vi "ME_acquire_8.vi"() -> ()   [LabVIEW 2015]
doc: "Use this template to build a producer/consumer design pattern. Use this template when you need to execute a process, such as data analysis, when a data source, such as a triggered acquisition, produces data at an uneven rate and you need to execute the process when the data becomes available."
uses:
  Mode.ctl
  oxford_driver/Oxford Drivers/BUSGEN.LLB/OxfordAddress.ctl
  <vilib>/Analysis/baseanly.llb/Mean (DBL).vi
  <vilib>/Utility/file.llb/Write Delimited Spreadsheet (DBL).vi
  <vilib>/express/express arith-compare/Formula/XNode/ExpressFormulaBlockNode.xnode
  <vilib>/Analysis/NI_AALBase.lvlib
panel:
  in  "Target Cnt":i8
  in  "Stop":bool
  out "SaveSweep":bool=TRUE
  out "Measurement File_dn":path
  out "Measurement File_up":path
  out "Measurement File_average":path
  out "Actual Polarization":dbl
  in  "Reset IB?":bool
  in  "First?":bool
  in  "Save Period":dbl=1.0
  out "Averaged I(B)":dbl[][](array[numeric])
  out "P(uC/mm^2)":dbl[](array[numeric])
  in  "Sweep Field":bool
  out "P(B)":cluster{"yi":dbl[], dbl[]}(graph)
  out "Offset array":dbl[](array[numeric])
  in  "stop 2":bool
  in  "dB":dbl=0.005
  in  "Dwell Time (ms)":u32=1
  out "appended array":dbl[][](array[numeric])
  in  "Magnet ON?":bool
  out "Actual B Field (T)":dbl
  out "Actual Temperature (K)":dbl
  out "Actual Current (pA)":dbl
  in  "Tab Control":T1(tab)
  out "P(T)":cluster{"yi":dbl[], dbl[]}(graph)
  out "I(T)":cluster{dbl[], dbl[]}(graph)
  in  "Set temperature (K)":dbl=4.5
  in  "Temp Ramping Rate (K/min)":dbl=10.0
  in  "Heater Range":enum16{"Off", "Low", "Medium", "High"}(ring)
  in  "Heater On/Off":bool
  in  "Sweep Rate Array":dbl[](array[numeric])=[2.0, 1.0, 0.5, 0.1, 0.05, 9.0, 10.0, 11.0, 12.0]
  out "I(B) 3":cluster{dbl[], dbl[]}[](graph)
  in  "Go to Set":bool
  in  "Set Field (T)":dbl=0.3
  in  "Field To Zero":bool
  in  "Sweep Rate (T/min)":dbl=2.0 format="%.6f"
  in  "Min Field (T)":dbl
  in  "Max Field (T)":dbl
  out "Up/Down":bool
  out "I(B) /Averaged/ 2":cluster{"B array":dbl[], dbl[]}[](graph)
  in  "Temperature Array":dbl[](array[numeric])=[4.5, 5.0, 6.0, 7.0, 8.0, 9.0, 10.0, 11.0, 12.0]
  in  "Measure Noise":bool
  in  "Cycles":i32
  in  "maximum value":dbl=10.0 format="%0.2f"
  in  "minimum value":dbl=-10.0 format="%0.2f"
  in  "physical channels":tag="Dev1/ai1"
  out "PSD (pA/Hz^1/2) Peaks Removed":cluster{"f0":dbl, "df":dbl, "magnitude":dbl[]}(graph)
  out "PSD (pA/Hz^1/2)":cluster{"f0":dbl, "df":dbl, "magnitude":dbl[]}(graph)
  out "Current (pA) Filtered":waveform(dbl)(graph)
  out "Current (pA)":dbl[](graph)
  in  "Samples per channel":i32=1000
  in  "Rate":dbl=1000.0 format="%0.2f"
  in  "Cut-Off Frequency":dbl=100.0 caption="Lower Cut-Off"
  in  "Filter On":bool
  out "Dc offset":dbl
  in  "Calibrate":bool
  in  "IV converter":refnum<visa-resource-name>="GPIB0::20::INSTR"
  in  "Magnetic Field":refnum<visa-resource-name>="GPIB0::21::INSTR"
  out "Time Lag":dbl=0.0500025749206543
  in  "Lake Shore":refnum<visa-resource-name>="GPIB0::11::INSTR"
  in  "Temp Refresh (s)":dbl=1.0
  in  "Sampling rate (Hz)":dbl=10.0
  in  "Gain (V/A)":dbl=1000000000.0
  in  "Sample area (mm^2)":dbl=3.9
  out "B_V":cluster{dbl[], "Best Linear Fit":dbl[]}[](graph)=[{[-0.00854253601, 0.00626134724, 0.0219834428, 0.0379117736, 0.0535871506, 0.0694316728, 0.0851615152, 0.100816481, 0.116478038, 0.132148461, 0.147876163, 0.16341701, 0.178976744, 0.194563632, 0.210251739, 0.225738944, 0.241298253, 0.256806034, 0.272344374, 0.287933477, 0.303494709, 0.318997125, 0.334591297, 0.350146681, 0.365618053, 0.380940961, 0.39666457, 0.412213675, 0.427724671, 0.443221444, 0.458760641, 0.474360042, 0.489915118, 0.505330598, 0.520967119, 0.536347531, 0.551813711, 0.567441155, 0.582995861, 0.598507522, 0.614041988, 0.629563151, 0.645106262, 0.660611914, 0.676136149, 0.691553948, 0.7071244, 0.72262999, 0.738171137, 0.753700392, 0.76919513, 0.784778028, 0.800215944, 0.8156961, 0.831325434, 0.846852183, 0.862326812, 0.877819169, 0.893312568, 0.90888536, 0.924354789], "Best Linear Fit"=[0.0, 0.005, 0.01, 0.015, 0.02, 0.025, 0.03, 0.035, 0.04, 0.045, 0.05, 0.055, 0.06, 0.065, 0.07, 0.075, 0.08, 0.085, 0.09, 0.095, 0.1, 0.105, 0.11, 0.115, 0.12, 0.125, 0.13, 0.135, 0.14, 0.145, 0.15, 0.155, 0.16, 0.165, 0.17, 0.175, 0.18, 0.185, 0.19, 0.195, 0.2, 0.205, 0.21, 0.215, 0.22, 0.225, 0.23, 0.235, 0.24, 0.245, 0.25, 0.255, 0.26, 0.265, 0.27, 0.275, 0.28, 0.285, 0.29, 0.295, 0.3]}, {[-0.00854253601, 0.00626134724, 0.0219834428, 0.0379117736, 0.0535871506, 0.0694316728, 0.0851615152, 0.100816481, 0.116478038, 0.132148461, 0.147876163, 0.16341701, 0.178976744, 0.194563632, 0.210251739, 0.225738944, 0.241298253, 0.256806034, 0.272344374, 0.287933477, 0.303494709, 0.318997125, 0.334591297, 0.350146681, 0.365618053, 0.380940961, 0.39666457, 0.412213675, 0.427724671, 0.443221444, 0.458760641, 0.474360042, 0.489915118, 0.505330598, 0.520967119, 0.536347531, 0.551813711, 0.567441155, 0.582995861, 0.598507522, 0.614041988, 0.629563151, 0.645106262, 0.660611914, 0.676136149, 0.691553948, 0.7071244, 0.72262999, 0.738171137, 0.753700392, 0.76919513, 0.784778028, 0.800215944, 0.8156961, 0.831325434, 0.846852183, 0.862326812, 0.877819169, 0.893312568, 0.90888536, 0.924354789], "Best Linear Fit"=[-0.00022554388023060128, 0.004536267537808887, 0.009593430775915074, 0.014716931562355689, 0.01975906732634002, 0.024855610270593523, 0.029915265354287977, 0.03495083565949541, 0.03998852608757118, 0.045029068349812316, 0.05008803495326229, 0.055086897848955874, 0.060091835929837946, 0.06510550835596321, 0.07015173884687344, 0.07513334727738563, 0.08013814865293042, 0.08512637555172443, 0.0901244320467579, 0.09513881694893507, 0.10014423687592358, 0.10513073807087174, 0.11014675346564809, 0.1151502923271957, 0.12012680792099008, 0.1250555686413888, 0.1301132186920259, 0.13511473785283767, 0.14010399888730068, 0.14508868495702945, 0.1500870171143548, 0.15510471446726903, 0.16010815425765457, 0.16506669165212906, 0.17009632901003072, 0.1750435864450521, 0.18001843198211442, 0.1850451496356715, 0.19004847041199868, 0.1950379453501071, 0.20003475573578386, 0.20502728708357412, 0.21002687821664084, 0.21501442030211, 0.220007939788244, 0.2249672231113706, 0.22997560874002893, 0.23496313088260184, 0.23996209027618054, 0.24495722449359253, 0.24994125598600042, 0.2549536449902534, 0.25991939913989753, 0.2648987401917687, 0.26992606578200207, 0.2749203939204135, 0.2798979571595809, 0.2848812227804405, 0.2898648235706211, 0.2948739618827834, 0.2998498524919418]}]
  out "V_I":cluster{dbl[], "Best Linear Fit":dbl[]}[](graph)=[{[0.0, 0.035, 0.069, 0.104, 0.138, 0.173, 0.208, 0.242, 0.277, 0.311, 0.346, 0.38, 0.415, 0.45, 0.484, 0.519, 0.553, 0.588, 0.623, 0.657, 0.692, 0.726, 0.761, 0.796, 0.83, 0.865, 0.899, 0.934, 0.969, 1.003, 1.038, 1.072, 1.107, 1.141, 1.176, 1.211, 1.245, 1.28, 1.314, 1.349, 1.384, 1.418, 1.453, 1.487, 1.522, 1.557, 1.591, 1.626, 1.66, 1.695, 1.73, 1.764, 1.799, 1.833, 1.868, 1.902, 1.937, 1.972, 2.006, 2.041, 2.075], "Best Linear Fit"=[-0.00854253601, 0.00626134724, 0.0219834428, 0.0379117736, 0.0535871506, 0.0694316728, 0.0851615152, 0.100816481, 0.116478038, 0.132148461, 0.147876163, 0.16341701, 0.178976744, 0.194563632, 0.210251739, 0.225738944, 0.241298253, 0.256806034, 0.272344374, 0.287933477, 0.303494709, 0.318997125, 0.334591297, 0.350146681, 0.365618053, 0.380940961, 0.39666457, 0.412213675, 0.427724671, 0.443221444, 0.458760641, 0.474360042, 0.489915118, 0.505330598, 0.520967119, 0.536347531, 0.551813711, 0.567441155, 0.582995861, 0.598507522, 0.614041988, 0.629563151, 0.645106262, 0.660611914, 0.676136149, 0.691553948, 0.7071244, 0.72262999, 0.738171137, 0.753700392, 0.76919513, 0.784778028, 0.800215944, 0.8156961, 0.831325434, 0.846852183, 0.862326812, 0.877819169, 0.893312568, 0.90888536, 0.924354789]}, {[0.0, 0.035, 0.069, 0.104, 0.138, 0.173, 0.208, 0.242, 0.277, 0.311, 0.346, 0.38, 0.415, 0.45, 0.484, 0.519, 0.553, 0.588, 0.623, 0.657, 0.692, 0.726, 0.761, 0.796, 0.83, 0.865, 0.899, 0.934, 0.969, 1.003, 1.038, 1.072, 1.107, 1.141, 1.176, 1.211, 1.245, 1.28, 1.314, 1.349, 1.384, 1.418, 1.453, 1.487, 1.522, 1.557, 1.591, 1.626, 1.66, 1.695, 1.73, 1.764, 1.799, 1.833, 1.868, 1.902, 1.937, 1.972, 2.006, 2.041, 2.075], "Best Linear Fit"=[-0.007846580254753975, 0.007882153481927697, 0.02316149482613275, 0.03889022856281441, 0.054169569907019474, 0.06989830364370113, 0.08562703738038281, 0.10090637872458785, 0.11663511246126955, 0.1319144538054746, 0.14764318754215625, 0.1629225288863613, 0.17865126262304296, 0.19437999635972467, 0.2096593377039297, 0.22538807144061138, 0.24066741278481643, 0.25639614652149806, 0.27212488025817977, 0.2874042216023848, 0.3031329553390665, 0.31841229668327153, 0.3341410304199532, 0.3498697641566349, 0.3651491055008399, 0.3808778392375216, 0.39615718058172666, 0.4118859143184083, 0.42761464805509, 0.442893989399295, 0.45862272313597674, 0.4739020644801818, 0.48963079821686345, 0.5049101395610684, 0.5206388732977502, 0.5363676070344319, 0.5516469483786369, 0.5673756821153185, 0.5826550234595236, 0.5983837571962053, 0.6141124909328869, 0.629391832277092, 0.6451205660137737, 0.6603999073579787, 0.6761286410946604, 0.691857374831342, 0.7071367161755471, 0.7228654499122288, 0.7381447912564338, 0.7538735249931156, 0.7696022587297972, 0.7848816000740022, 0.8006103338106839, 0.815889675154889, 0.8316184088915707, 0.8468977502357756, 0.8626264839724573, 0.878355217709139, 0.893634559053344, 0.9093632927900257, 0.9246426341342309]}]
  out "B0 (T)":dbl=0.0025222449819540214
  out "B/V (T/V)":dbl=0.321659617116981
  out "I0 (A)":dbl=-0.007846580254753975
  out "V/I (Ohm)":dbl=0.44939239247661916
  in  "Offset?":bool
  in  "Temp/Magnetic Field":bool
  out "index":i8
  out "Read?":bool
  out "Magnetic Field (T)":dbl[](array[numeric])
  out "Reset":bool
  out "Measured Current (pA)":dbl[](array[numeric])
  out "Elapsed Time (s)":dbl[](array[numeric])
  out "Start time":timestamp
  in  "Enum":T2=enum."Process"
  out "B array":dbl[](array[numeric])
  in  "dB (T)":dbl=0.005
  in  "Counter":i8
  out "L magnet (H)":dbl
  out "R magnet (mOhm)":dbl
  out "Actual Current (R0)":dbl
  out "Actual Field (T)":dbl
  out "Temperature array":dbl[](array[numeric])
  in  "New Measurement File":bool
  out "Measurement File":path
  out "refnum out":refnum<file>
  in  "Measuring":bool
  in  "Measure /Pause":bool
  in  "stop":bool
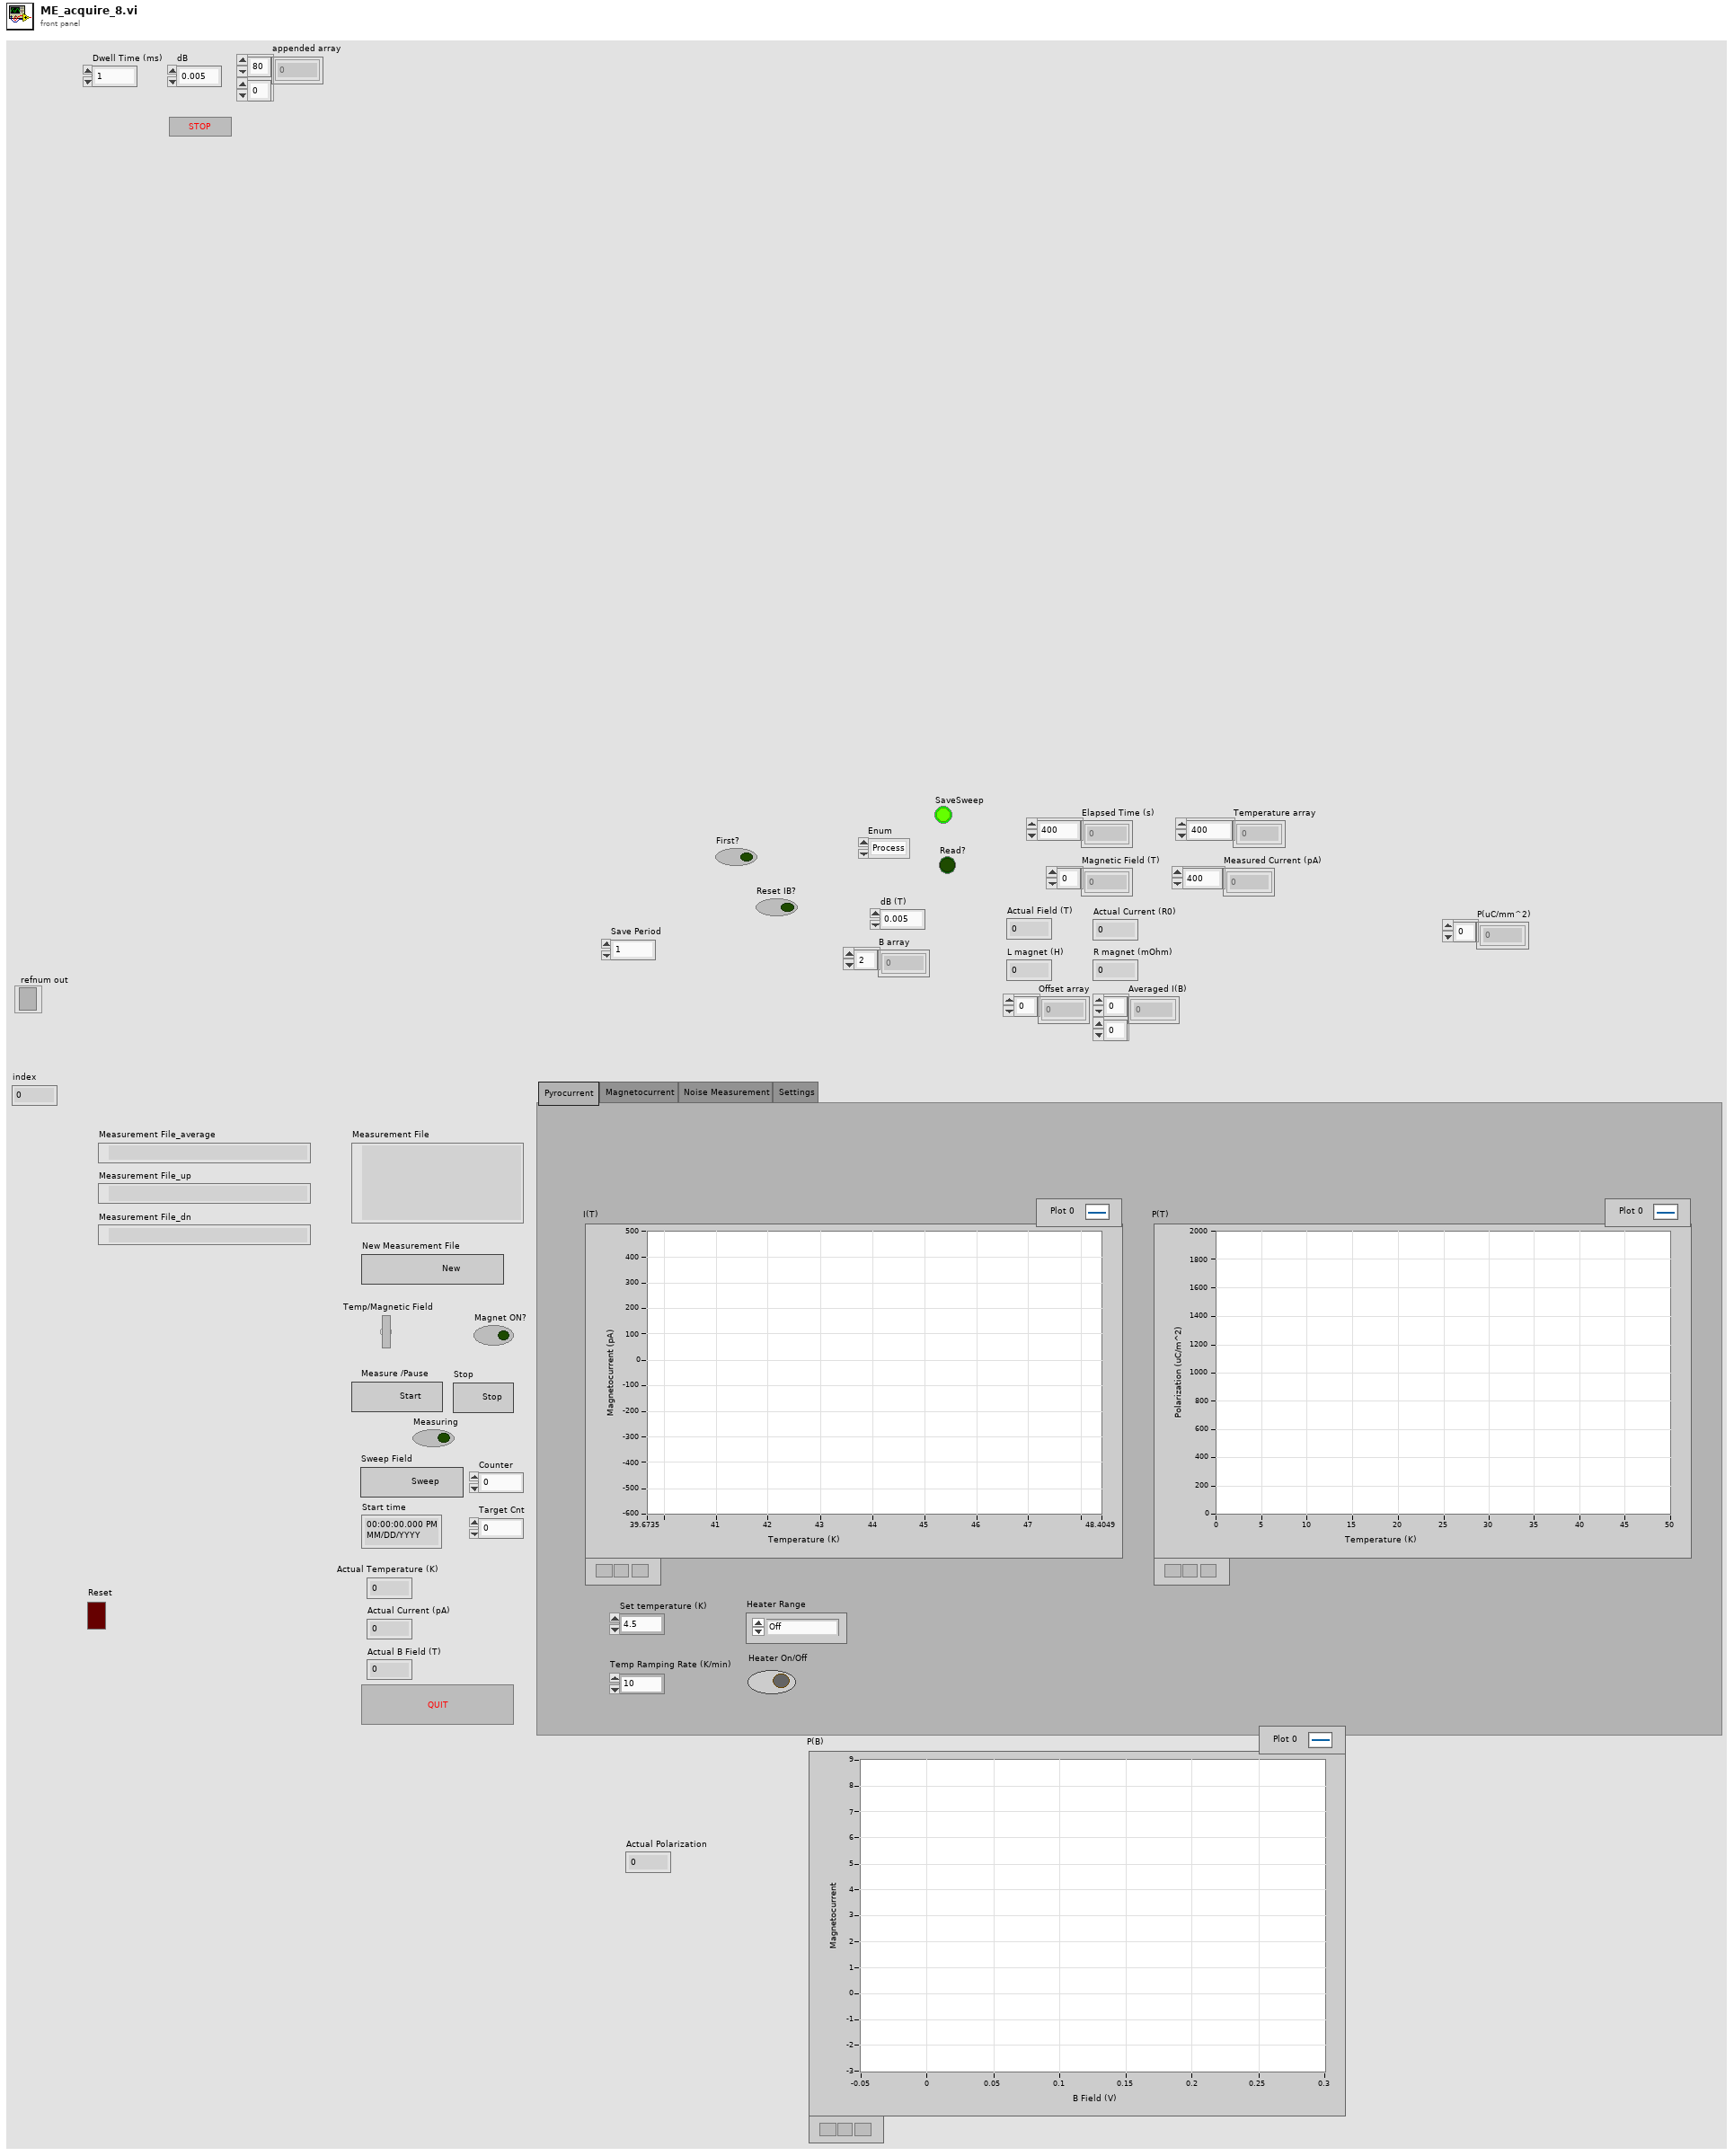
[diagram p1: front panel]
types:
  T1 = enum32{"Pyrocurrent", "Magnetocurrent", "Noise Measurement", "Settings"}
  T2 = typedef "Mode.ctl" = enum16{"Offset", "Process", "Sweep", "Plot", "Save", "New"}
  T3 = enum16{"open", "replace", "create", "open or create", "replace or create", "replace or create with confirmation"}
  T4 = typedef "OxfordAddress.ctl" = cluster{"Com Port":i32, "ISOBUS Address":i32, "GPIB Address":i16, "Communication":enum16{"RS232", "ISOBUS", "GPIB", "Gateway"}}
  T5 = cluster{"seconds since 1Jan1904":timestamp, "read buffer":string, "read buffer":string}
  T6 = cluster{"B array":dbl[], "Averaged I(B) out":dbl[]}
  T7 = cluster{"B array":dbl[], "Averaged I(B) out":dbl[]}[]
  T8 = cluster{"I array out (A)":dbl[], "V array out (V)":dbl[]}
  T9 = cluster{"I array out (A)":dbl[], "Best Linear Fit":dbl[]}
  T10 = cluster{"V array out (V)":dbl[], "B array Out":dbl[]}
  T11 = cluster{"V array out (V)":dbl[], "Best Linear Fit 2":dbl[]}
  T12 = cluster{"I array out (A)":dbl[], "Best Linear Fit":dbl[]}[]
  T13 = cluster{"V array out (V)":dbl[], "Best Linear Fit 2":dbl[]}[]
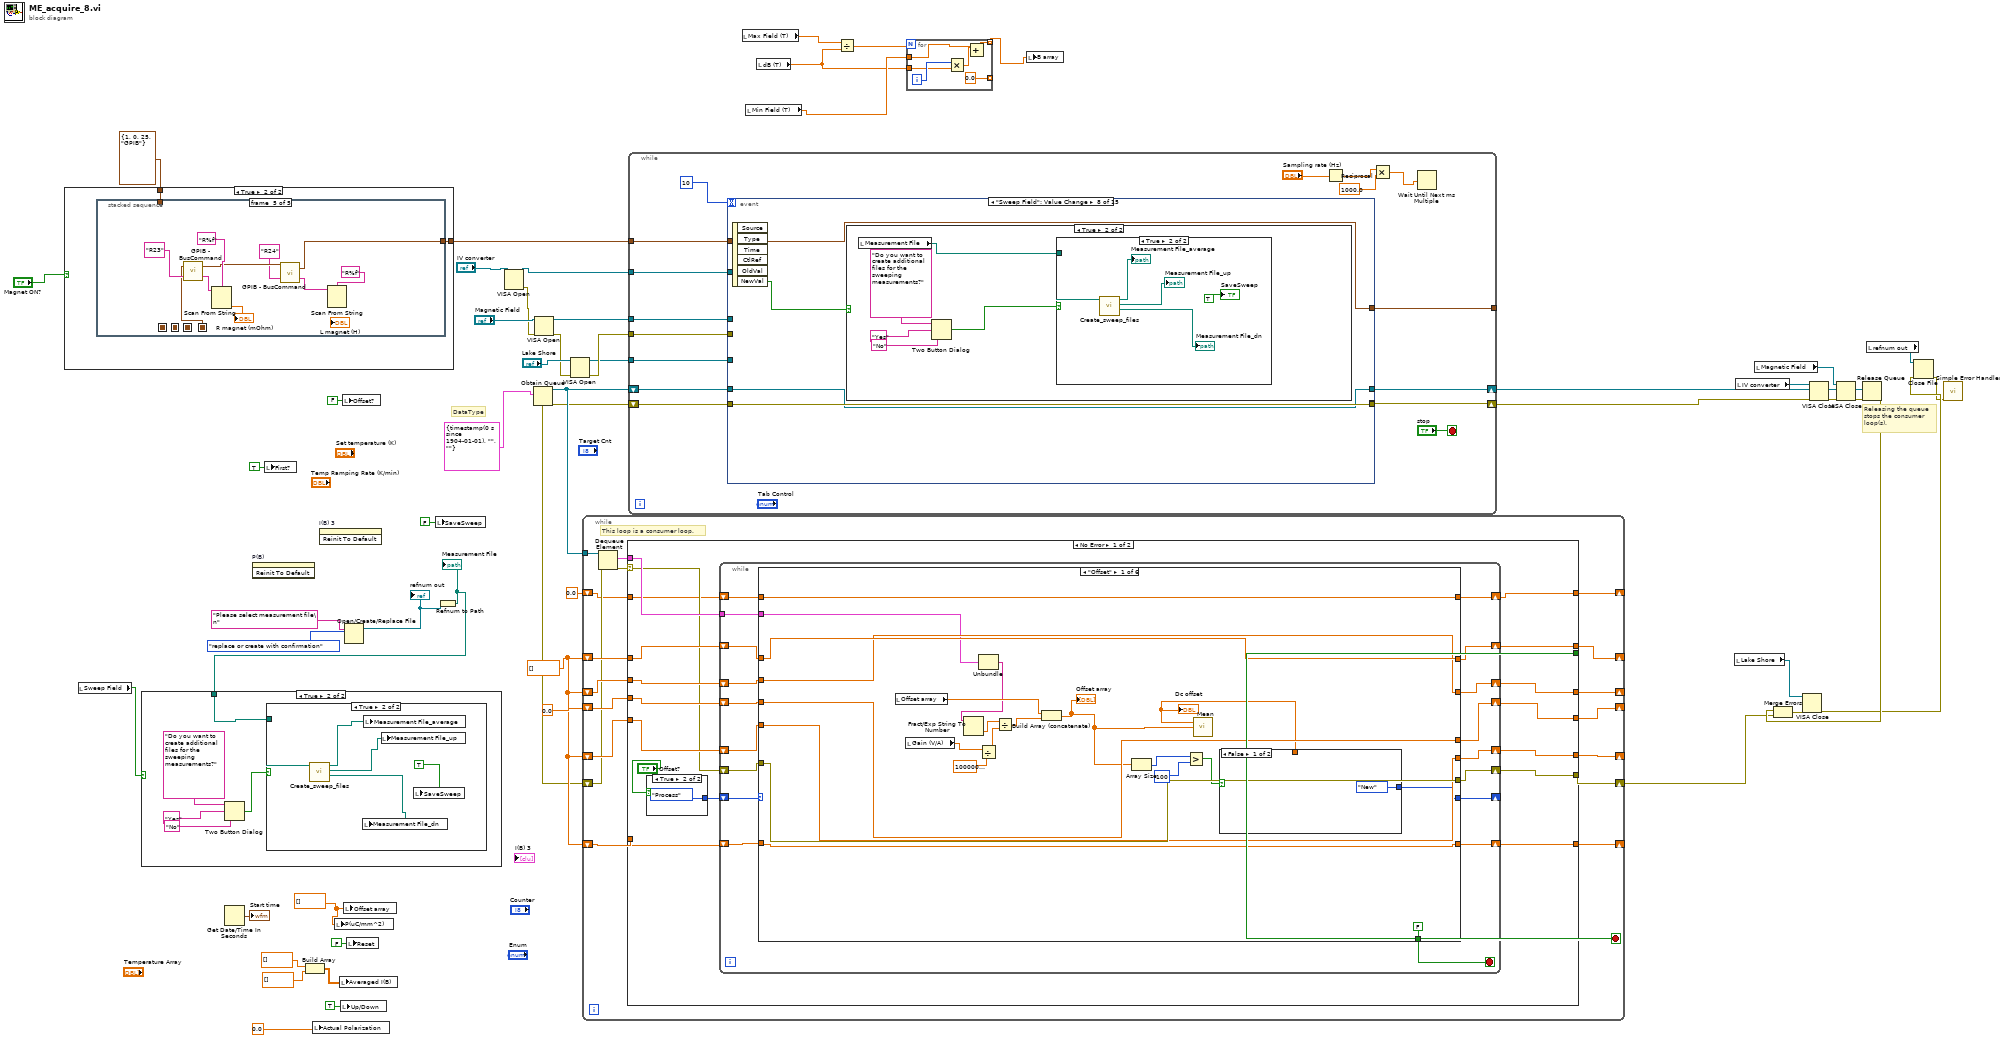
[diagram p0: block diagram]
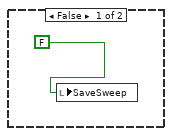
[diagram p3: hidden frame]
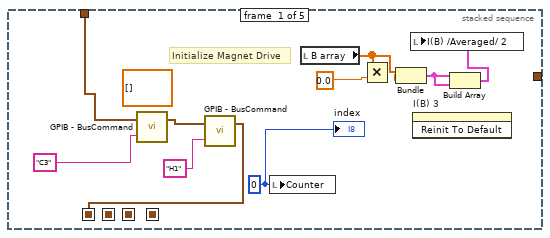
[diagram p5: hidden frame]
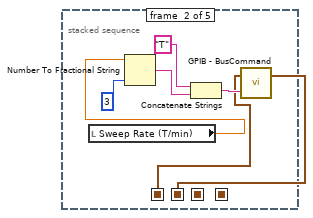
[diagram p6: hidden frame]
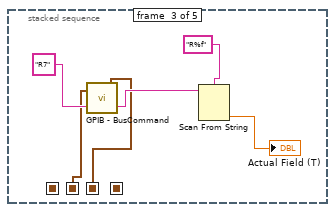
[diagram p7: hidden frame]
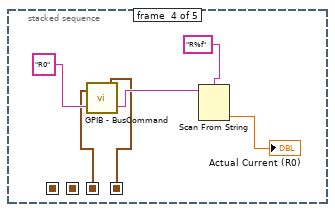
[diagram p8: hidden frame]
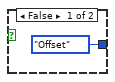
[diagram p9: hidden frame]
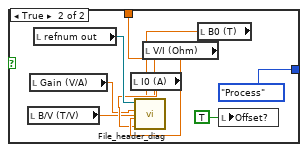
[diagram p10: hidden frame]
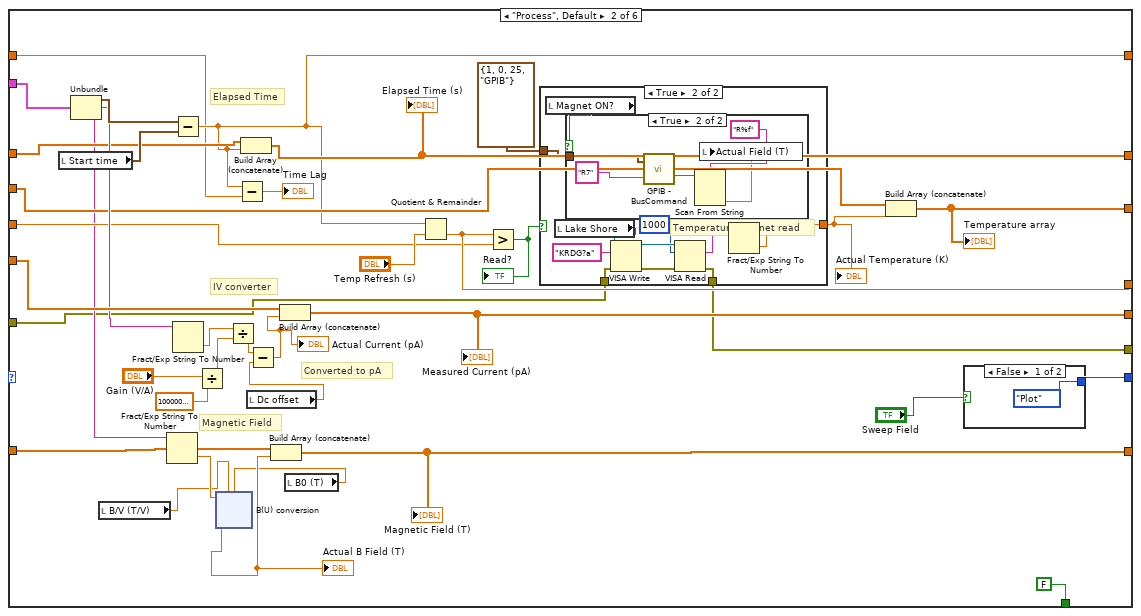
[diagram p11: hidden frame]
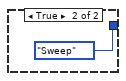
[diagram p12: hidden frame]
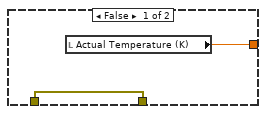
[diagram p13: hidden frame]
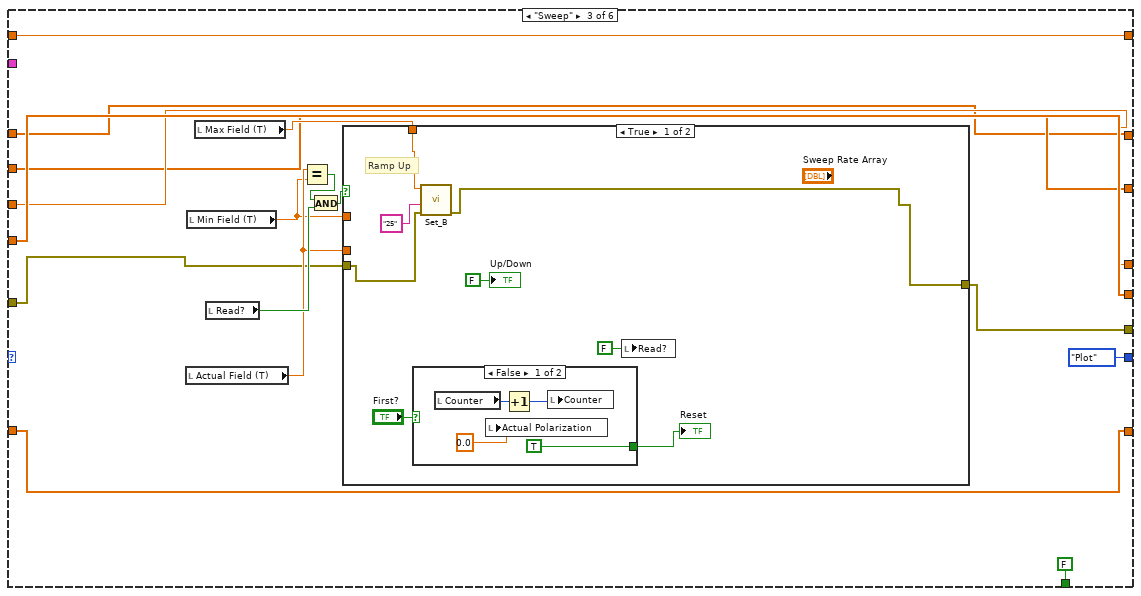
[diagram p15: hidden frame]
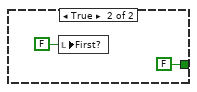
[diagram p16: hidden frame]
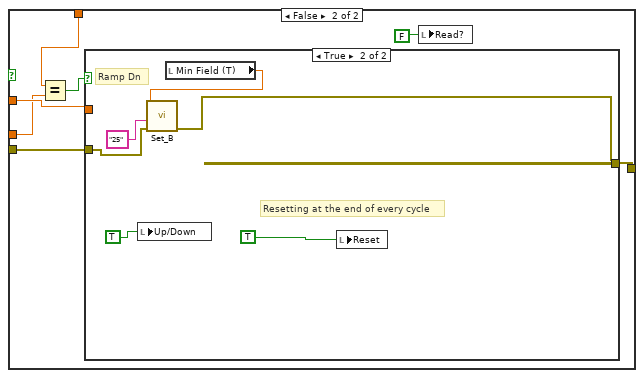
[diagram p17: hidden frame]
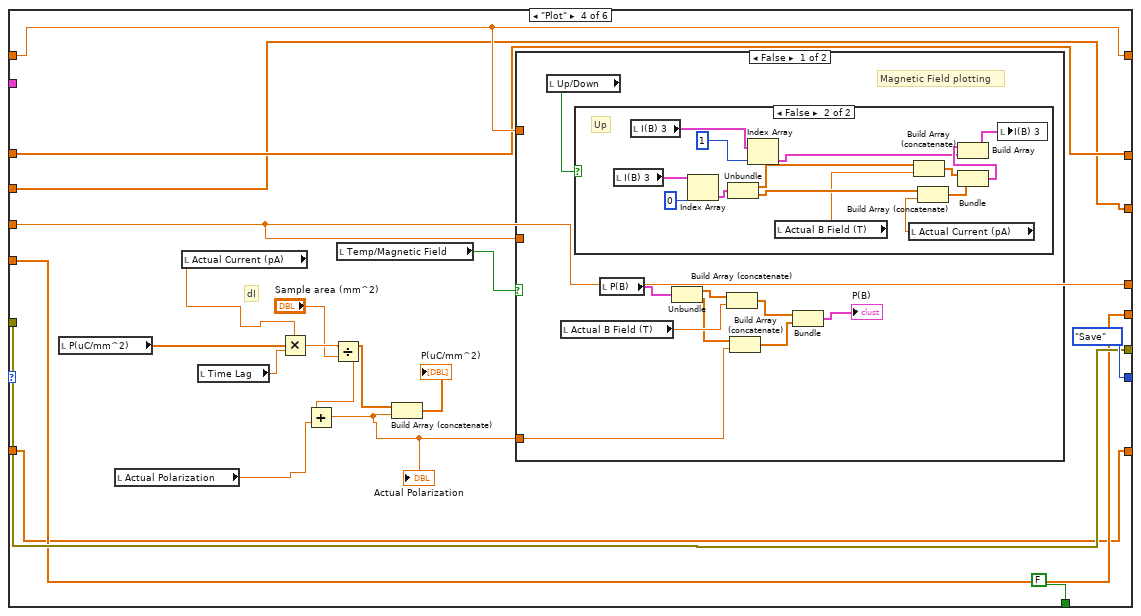
[diagram p19: hidden frame]
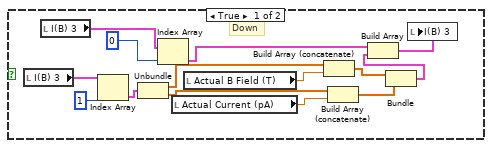
[diagram p20: hidden frame]
diagram:
  w16 = dbl[] []
  w23 = dbl[] []
  # "DataType"
  # "Releasing the queue stops the consumer loop(s)."
  n1 = case shown="True" "Magnet ON?" {
    tunnel: T4 {"Com Port"=1, "ISOBUS Address"=0, "GPIB Address"=25, "Communication"=enum."GPIB"} ("Address") -> [w53 w55]
    tunnel: [w53 w54] -> w31
    frame False {
    }
    frame True {
      n2 = stacked-sequence {
        seq-local: [w63 _ _ _ _] -> [_ w68 _ _ _]
        seq-local: [_ w67 _ _ _] -> [_ _ w75 _ _]
        seq-local: [_ _ w74 _ _] -> [_ _ _ w81 _]
        seq-local: [_ _ _ w80 _] -> [_ _ _ _ w91]
        tunnel: w55 -> [w65 _ _ _ _]
        tunnel: [_ _ _ _ w89] -> w54
        frame #0 {
          (unwired) dbl[][] []
          w61 = i8 0 ("Counter")
          # "Initialize Magnet Drive"
          n3 = call "GPIB - BusCommand.vi"("Command"="C3", "Address"=w65) -> ("Address(thru)"=w64:T4)  [unwired: 1 out]
          n4 = call "GPIB - BusCommand.vi"("Command"="H1", "Address"=w64) -> ("Address(thru)"=w63:T4)  [unwired: 1 out]
          n5 = local write "Counter"(w61) -> ()
          n6 = local read "B array"() -> (w59:dbl[])
          n7 = Multiply(x=w59, y=0.0) -> (x*y=w58:dbl[])
          n8 = Bundle("B array"=w59, w58) -> (w57:cluster{"B array":dbl[], dbl[]})  [unwired: 1 in]
          n9 = invoke on="I(B) 3" class="XYGraph (strict)" method="Reinit To Default"() -> ()  [unwired: 3 in, 3 out]
          n10 = Build Array(w57, w57) -> (w56:cluster{"B array":dbl[], dbl[]}[])
          n11 = local write "I(B) /Averaged/ 2"(w56) -> ()
          "index" <- w61
        }
        frame #1 {
          n12 = local read "Sweep Rate (T/min)"() -> (w69:dbl)
          n13 = Number To Fractional String(number=w69, precision (6)=i16 3) -> (F-format string=w71:string)  [unwired: 2 in]
          n14 = Concatenate Strings("T" ("format string"), w71) -> (w70:string)
          n15 = call "GPIB - BusCommand.vi"("Command"=w70, "Address"=w68) -> ("Address(thru)"=w67:T4)  [unwired: 1 out]
        }
        frame #2 {
          n16 = call "GPIB - BusCommand.vi"("Command"="R7" ("format string"), "Address"=w75) -> ("Reply"=w79:string, "Address(thru)"=w74:T4)
          n17 = Scan From String(format string="R%f" ("remaining string"), input string=w79) -> (output 1=→"Actual Field (T)":dbl)  [unwired: 3 in, 3 out]
        }
        frame #3 {
          n18 = call "GPIB - BusCommand.vi"("Command"="R0" ("format string"), "Address"=w81) -> ("Reply"=w85:string, "Address(thru)"=w80:T4)
          n19 = Scan From String(format string="R%f" ("remaining string"), input string=w85) -> (output 1=→"Actual Current (R0)":dbl)  [unwired: 3 in, 3 out]
        }
        frame #4 {
          n20 = call "GPIB - BusCommand.vi"("Command"="R23" ("format string"), "Address"=w91) -> ("Reply"=w95:string, "Address(thru)"=w90:T4)
          n21 = Scan From String(format string="R%f" ("remaining string"), input string=w95) -> (output 1=→"R magnet (mOhm)":dbl)  [unwired: 3 in, 3 out]
          n22 = call "GPIB - BusCommand.vi"("Command"="R24" ("format string"), "Address"=w90) -> ("Reply"=w87:string, "Address(thru)"=w89:T4)
          n23 = Scan From String(format string="R%f" ("remaining string"), input string=w87) -> ()  [unwired: 4 in, 3 out]
        }
      }
    }
  }
  n24 = local read "Sweep Field"() -> (w2:bool)
  n25 = Get Date/Time In Seconds() -> (seconds since 1Jan1904=→"Start time":timestamp)
  n26 = invoke on="P(B)" class="XYGraph (strict)" method="Reinit To Default"() -> ()  [unwired: 3 in, 3 out]
  n27 = local write "First?"(TRUE ("First?")) -> ()
  n28 = Build Array(dbl[] [], dbl[] []) -> (w13:dbl[][])
  n29 = local write "Actual Polarization"(0.0 ("Actual Polarization")) -> ()
  n30 = invoke on="I(B) 3" class="XYGraph (strict)" method="Reinit To Default"() -> ()  [unwired: 3 in, 3 out]
  n31 = local write "P(uC/mm^2)"(w16) -> ()
  n32 = local write "Averaged I(B)"(w13) -> ()
  n33 = local write "Up/Down"(TRUE ("Up/Down")) -> ()
  n34 = local write "Offset?"(FALSE ("Offset?")) -> ()
  n35 = local write "Offset array"(w16) -> ()
  n36 = Open/Create/Replace File(prompt="Please select measurement file\n", operation (0:open)=T3."replace or create with confirmation") -> (refnum out=w28:refnum<file>)  [unwired: 4 in, 2 out]
  "refnum out" <- w28
  n37 = local write "Reset"(FALSE ("Reset")) -> ()
  n38 = local write "SaveSweep"(FALSE ("SaveSweep")) -> ()
  n39 = Refnum to Path(1:w28) -> (0:w1:path)
  "Measurement File" <- w1
  n40 = case shown="True" w2 {
    tunnel: w1 -> [_ w96]
    frame False {
    }
    frame True {
      n41 = Two Button Dialog(message="Do you want to create additional files for the sweeping measurements?" ("string"), 1:"No" ("F button name (\"Cancel\")"), 2:"Yes" ("T button name (\"OK\")")) -> (T button?=w98:bool)
      n42 = case shown="True" w98 {
        tunnel: w96 -> [_ w106]
        frame False {
          n43 = local write "SaveSweep"(FALSE ("SaveSweep")) -> ()
        }
        frame True {
          n44 = call "Create_sweep_files.vi"("Measurement File"=w106) -> ("Path 3"=w103:path, "Path 2"=w104:path, "Path"=w105:path)  [unwired: 8 in]
          n45 = local write "Measurement File_dn"(w103) -> ()
          n46 = local write "Measurement File_average"(w105) -> ()
          n47 = local write "Measurement File_up"(w104) -> ()
          n48 = local write "SaveSweep"(TRUE) -> ()
        }
      }
    }
  }
  n49 = VISA Open(VISA resource name="IV converter") -> (VISA resource name=w47:refnum<visa-resource-name>, error out=w49:errorcluster)  [unwired: 4 in]
  n50 = Obtain Queue(element data type=T5 {"seconds since 1Jan1904"=timestamp(0 s since 1904-01-01), "read buffer"="", "read buffer"=""} ("output cluster")) -> (queue out=w52:refnum<queue>, error out=w21:errorcluster)  [unwired: 4 in, 1 out]
  n51 = VISA Open(error in (no error)=w49, VISA resource name="Magnetic Field") -> (VISA resource name=w46:refnum<visa-resource-name>, error out=w25:errorcluster)  [unwired: 3 in]
  n52 = VISA Open(error in (no error)=w25, VISA resource name="Lake Shore") -> (VISA resource name=w19:refnum<visa-resource-name>, error out=w24:errorcluster)  [unwired: 3 in]
  n53 = while {
    tunnel: w52 -> [w124]
    shift-right: [w119] -> _
    shift-left: w23 -> [w118]
    shift-right: [w117] -> _
    shift-left: w23 -> [w116]
    shift-right: [w115] -> _
    shift-left: w23 -> [w114]
    shift-right: [w113] -> _
    shift-left: 0.0 -> [w112]
    shift-right: [w111] -> _
    shift-left: w23 -> [w110]
    shift-right: [w120] -> w36
    shift-left: w21 -> [w109]
    shift-right: [w108] -> _
    shift-left: 0.0 -> [w107]
    stop <- w121 stop-if-true
    # "This loop is a consumer loop."
    n54 = Dequeue Element(queue=w124, error in (no error)=w109) -> (element=w122:T5, error out=w123:errorcluster)  [unwired: 1 in, 2 out]
    n55 = case shown="No Error" w123 {
      selector: w123 -> [w129 w462]
      tunnel: w122 -> [w140 _]
      tunnel: [_ TRUE] -> w121
      tunnel: [w128 w462] -> w120
      tunnel: [w139 w461] -> w119
      tunnel: w118 -> [w138 w461]
      tunnel: [w137 w458] -> w117
      tunnel: w116 -> [w136 w458]
      tunnel: [w135 w457] -> w115
      tunnel: w114 -> [w134 w457]
      tunnel: [w133 w459] -> w113
      tunnel: w112 -> [w132 w459]
      tunnel: [w131 w460] -> w111
      tunnel: w110 -> [w130 w460]
      tunnel: [w127 w456] -> w108
      tunnel: w107 -> [w126 w456]
      frame No Error {
        n56 = case shown="True" "Offset?" {
          tunnel: [Mode."Offset" ("Enum") Mode."Process" ("Enum")] -> w141
          frame False {
          }
          frame True {
          }
        }
        n57 = while {
          shift-right: [w149] -> _
          shift-left: w141 -> [w161]
          tunnel: w140 -> [w160]
          shift-right: [w159] -> w139
          shift-left: w138 -> [w158]
          shift-right: [w151] -> w131
          shift-left: w130 -> [w150]
          shift-right: [w153] -> w133
          shift-left: w132 -> [w152]
          shift-right: [w157] -> w137
          shift-left: w136 -> [w156]
          shift-right: [w147] -> w128
          shift-left: w129 -> [w148]
          shift-right: [w155] -> w135
          shift-left: w134 -> [w154]
          shift-right: [w145] -> w127
          shift-left: w126 -> [w144]
          stop <- w146 stop-if-true
          n58 = case shown="\"Offset\"" w161 {
            tunnel: w160 -> [w176 w229 _ _ _ _]
            tunnel: [w183 w226 w266 w319 w392 w454] -> w159
            tunnel: w158 -> [w183 w217 w266 w319 w388 w454]
            tunnel: [w177 w225 w269 w321 w394 w451] -> w157
            tunnel: w156 -> [w177 w224 w269 w321 w389 w451]
            tunnel: [w179 w221 w271 w316 w395 w448] -> w155
            tunnel: w154 -> [w179 w220 w271 w316 w390 w448]
            tunnel: [w181 w216 w268 w317 w398 w452] -> w153
            tunnel: w152 -> [w181 w215 w268 w317 w398 w452]
            tunnel: [w182 w212 w267 w318 w393 w453] -> w151
            tunnel: w150 -> [w182 w213 w267 w318 w391 w453]
            tunnel: [w165 w210 Mode."Plot" ("Enum") Mode."Save" ("Enum") Mode."New" ("Enum") Mode."Process" ("Enum")] -> w149
            tunnel: w148 -> [w180 w208 w273 w324 w397 w450]
            tunnel: [w180 w207 w272 w324 w397 w450] -> w147
            tunnel: [FALSE FALSE FALSE FALSE FALSE TRUE] -> w146
            tunnel: [w164 w204 w265 w320 w396 w447] -> w145
            tunnel: w144 -> [w164 w203 w265 w320 w396 w447]
            frame "Offset" {
              n59 = local read "Offset array"() -> (w170:dbl[])
              n60 = local read "Gain (V/A)"() -> (w174:dbl)
              n61 = Unbundle(w176) -> ("read buffer"=w163:string)  [unwired: 2 out]
              n62 = Fract/Exp String To Number(string=w163) -> (number=w175:dbl)  [unwired: 3 in, 1 out]
              n63 = Divide(x=w174, y=1000000000000.0) -> (x/y=w172:dbl)
              n64 = Divide(x=w175, y=w172) -> (x/y=w171:dbl)
              n65 = Build Array (concatenate)(w170, w171) -> (w166:dbl[])
              "Offset array" <- w166
              n66 = Array Size(array=w166) -> (size(s)=w169:i32)
              n67 = Greater?(x=w169, y=100) -> (0:w167:bool)
              n68 = call-poly <vilib>:"Mean.vi"("X"=w166) -> ("mean"=w162:dbl)  [unwired: 1 out]
              "Dc offset" <- w162
              n69 = case shown="False" w167 {
                tunnel: [Mode."New" ("Enum") Mode."Process" ("Enum")] -> w165
                tunnel: w162 -> [_ w185]
                frame False {
                }
                frame True {
                  n70 = local read "B/V (T/V)"() -> (w186:dbl)
                  n71 = local read "Gain (V/A)"() -> (w187:dbl)
                  n72 = local read "refnum out"() -> (w191:refnum<file>)
                  n73 = local read "I0 (A)"() -> (w189:dbl)
                  n74 = local read "V/I (Ohm)"() -> (w190:dbl)
                  n75 = local read "B0 (T)"() -> (w188:dbl)
                  n76 = call "File_header_diag.vi"("OFFSET"=w185, "B0"=w188, "B/V"=w186, "I0"=w189, "V/I"=w190, "Gain"=w187, "Byte Stream File in"=w191) -> ()  [unwired: 5 in]
                  n77 = local write "Offset?"(TRUE ("Offset?")) -> ()
                }
              }
            }
            frame "Process", Default {
              # "Converted to pA"
              # "Magnetic Field"
              # "IV converter"
              # "Elapsed Time"
              n78 = local read "Start time"() -> (w227:timestamp)
              n79 = Unbundle(w229) -> ("seconds since 1Jan1904"=w228:timestamp, "read buffer"=w222:string, "read buffer"=w209:string)
              n80 = local read "B/V (T/V)"() -> (w199:dbl)
              n81 = Fract/Exp String To Number(string=w209) -> (number=w219:dbl)  [unwired: 3 in, 1 out]
              n82 = Subtract(x=w228, y=w227) -> (x-y=w204:dbl)
              n83 = Fract/Exp String To Number(string=w222) -> (number=w223:dbl)  [unwired: 3 in, 1 out]
              n84 = Divide(x="Gain (V/A)", y=1000000000000.0) -> (x/y=w202:dbl)
              n85 = Divide(x=w223, y=w202) -> (x/y=w197:dbl)
              n86 = Subtract(x=w204, y=w203) -> (x-y=→"Time Lag":dbl)
              n87 = Build Array (concatenate)(w217, w204) -> (w226:dbl[])
              "Elapsed Time (s)" <- w226
              n88 = local read "Dc offset"() -> (w195:dbl)
              n89 = Subtract(x=w197, y=w195) -> (x-y=w196:dbl)
              "Actual Current (pA)" <- w196
              n90 = Build Array (concatenate)(w224, w196) -> (w225:dbl[])
              "Measured Current (pA)" <- w225
              n91 = local read "B0 (T)"() -> (w198:dbl)
              n92 = xnode "B(U) conversion"("V"=w219, "BpV"=w199, "B0"=w198) -> ("Result"=w218:dbl)  [unwired: 1 in, 1 out]
              "Actual B Field (T)" <- w218
              n93 = Build Array (concatenate)(w220, w218) -> (w221:dbl[])
              "Magnetic Field (T)" <- w221
              n94 = Quotient & Remainder(x=w204, y="Temp Refresh (s)") -> (floor(x/y)=w216:dbl)  [unwired: 1 out]
              n95 = Greater?(x=w216, y=w215) -> (0:w214:bool)
              "Read?" <- w214
              n96 = case shown="True" w214 {
                tunnel: [w235 w241] -> w211
                tunnel: w208 -> [w234 w240]
                tunnel: [w234 w239] -> w207
                tunnel: T4 {"Com Port"=1, "ISOBUS Address"=0, "GPIB Address"=25, "Communication"=enum."GPIB"} ("Address") -> [_ w238]
                frame False {
                  n97 = local read "Actual Temperature (K)"() -> (w235:dbl)
                }
                frame True {
                  # "Temperature/Magnet read"
                  n98 = local read "Magnet ON?"() -> (w236:bool)
                  n99 = local read "Lake Shore"() -> (w237:refnum<visa-resource-name>)
                  n100 = case shown="True" w236 {
                    tunnel: w238 -> [_ w248]
                    frame False {
                    }
                    frame True {
                      n101 = call "GPIB - BusCommand.vi"("Command"="R7" ("format string"), "Address"=w248) -> ("Reply"=w249:string)  [unwired: 1 out]
                      n102 = Scan From String(format string="R%f" ("remaining string"), input string=w249) -> (output 1=w247:dbl)  [unwired: 3 in, 3 out]
                      n103 = local write "Actual Field (T)"(w247) -> ()
                    }
                  }
                  n104 = VISA Write(VISA resource name=w237, write buffer="KRDG?a", error in (no error)=w240) -> (VISA resource name out=w245:refnum<visa-resource-name>, error out=w244:errorcluster)  [unwired: 1 out]
                  n105 = VISA Read(VISA resource name=w245, byte count=u32 1000, error in (no error)=w244) -> (read buffer=w242:string, error out=w239:errorcluster)  [unwired: 2 out]
                  n106 = Fract/Exp String To Number(string=w242) -> (number=w241:dbl)  [unwired: 3 in, 1 out]
                }
              }
              "Actual Temperature (K)" <- w211
              n107 = Build Array (concatenate)(w213, w211) -> (w212:dbl[])
              "Temperature array" <- w212
              n108 = case shown="False" "Sweep Field" {
                tunnel: [Mode."Plot" ("Enum") Mode."Sweep" ("Enum")] -> w210
                frame False {
                }
                frame True {
                }
              }
            }
            frame "Sweep" {
              n109 = local read "Actual Field (T)"() -> (w276:dbl)
              n110 = local read "Min Field (T)"() -> (w275:dbl)
              n111 = local read "Max Field (T)"() -> (w274:dbl)
              n112 = local read "Read?"() -> (w279:bool)
              n113 = Equal?(x=w276, y=w275) -> (x = y?=w277:bool)
              n114 = And(x=w277, y=w279) -> (x .and. y?=w278:bool)
              n115 = case shown="True" w278 {
                tunnel: [w286 w300] -> w272
                tunnel: w274 -> [w287 w299]
                tunnel: w275 -> [_ w298]
                tunnel: w276 -> [_ w296]
                tunnel: w273 -> [w285 w295]
                frame True {
                  # "Ramp Up"
                  n116 = case shown="False" "First?" {
                    tunnel: [TRUE ("Save") FALSE ("Save")] -> w280
                    frame False {
                      n117 = local read "Counter"() -> (w290:i8)
                      n118 = local write "Actual Polarization"(0.0 ("Actual Polarization")) -> ()
                      n119 = Increment(x=w290) -> (x+1=w291:i8)
                      n120 = local write "Counter"(w291) -> ()
                    }
                    frame True {
                      n121 = local write "First?"(FALSE ("First?")) -> ()
                    }
                  }
                  "Reset" <- w280
                  n122 = call "Set_B.vi"("error in (no error)"=w285, "address string"="25", "Set Field (T)"=w287) -> ("error out"=w286:errorcluster)  [unwired: 8 in]
                  n123 = local write "Read?"(FALSE ("Read?")) -> ()
                  "Up/Down" <- FALSE ("Up/Down")
                }
                frame False {
                  n124 = Equal?(x=w299, y=w296) -> (x = y?=w297:bool)
                  n125 = case shown="True" w297 {
                    tunnel: [w301 w304] -> w300
                    tunnel: w298 -> [_ _]
                    tunnel: w295 -> [w301 w305]
                    frame False {
                    }
                    frame True {
                      # "Resetting at the end of every cycle"
                      # "Ramp Dn"
                      n126 = local write "Up/Down"(TRUE ("Up/Down")) -> ()
                      n127 = local read "Min Field (T)"() -> (w303:dbl)
                      n128 = call "Set_B.vi"("error in (no error)"=w305, "address string"="25", "Set Field (T)"=w303) -> ("error out"=w304:errorcluster)  [unwired: 8 in]
                      n129 = local write "Reset"(TRUE ("Reset")) -> ()
                    }
                  }
                  n130 = local write "Read?"(FALSE ("Read?")) -> ()
                }
              }
            }
            frame "Plot" {
              # "dI"
              n131 = local read "P(uC/mm^2)"() -> (w309:dbl[])
              n132 = local read "Actual Polarization"() -> (w308:dbl)
              n133 = local read "Actual Current (pA)"() -> (w310:dbl)
              n134 = local read "Time Lag"() -> (w322:dbl)
              n135 = Multiply(x=w310, y=w322) -> (x*y=w314:dbl)
              n136 = Divide(x=w314, y="Sample area (mm^2)") -> (x/y=w313:dbl)
              n137 = Add(x=w313, y=w308) -> (x+y=w312:dbl)
              "Actual Polarization" <- w312
              n138 = local read "Temp/Magnetic Field"() -> (w323:bool)
              n139 = Build Array (concatenate)(w309, w312) -> (→"P(uC/mm^2)":dbl[])
              n140 = case shown="False" w323 {
                tunnel: w320 -> [_ w383]
                tunnel: w317 -> [_ w381]
                tunnel: w312 -> [w330 w364]
                frame False {
                  # "Magnetic Field plotting"
                  n141 = local read "Up/Down"() -> (w335:bool)
                  n142 = local read "Actual B Field (T)"() -> (w332:dbl)
                  n143 = case shown="False" w335 {
                    frame True {
                      # "Down"
                      n144 = local read "I(B) 3"() -> (w345:cluster{dbl[], dbl[]}[])
                      n145 = local read "I(B) 3"() -> (w349:cluster{dbl[], dbl[]}[])
                      n146 = Index Array(array=w345, index=1) -> (element=w343:cluster{dbl[], dbl[]})
                      n147 = Unbundle(w343) -> (w342:dbl[], w341:dbl[])
                      n148 = Index Array(array=w349, index=i8 0 ("t")) -> (element=w346:cluster{dbl[], dbl[]})
                      n149 = local read "Actual Current (pA)"() -> (w338:dbl)
                      n150 = local read "Actual B Field (T)"() -> (w337:dbl)
                      n151 = Build Array (concatenate)(w342, w337) -> (w340:dbl[])
                      n152 = Build Array (concatenate)(w341, w338) -> (w339:dbl[])
                      n153 = Bundle(w340, w339) -> (w336:cluster{dbl[], dbl[]})  [unwired: 1 in]
                      n154 = Build Array(w346, w336) -> (w347:cluster{dbl[], dbl[]}[])
                      n155 = local write "I(B) 3"(w347) -> ()
                    }
                    frame False {
                      # "Up"
                      n156 = local read "I(B) 3"() -> (w361:cluster{dbl[], dbl[]}[])
                      n157 = local read "I(B) 3"() -> (w363:cluster{dbl[], dbl[]}[])
                      n158 = Index Array(array=w361, index=0) -> (element=w359:cluster{dbl[], dbl[]})
                      n159 = Unbundle(w359) -> (w358:dbl[], w357:dbl[])
                      n160 = Index Array(array=w363, index=i8 1 ("t")) -> (element=w351:cluster{dbl[], dbl[]})
                      n161 = local read "Actual B Field (T)"() -> (w353:dbl)
                      n162 = local read "Actual Current (pA)"() -> (w352:dbl)
                      n163 = Build Array (concatenate)(w358, w353) -> (w356:dbl[])
                      n164 = Build Array (concatenate)(w357, w352) -> (w355:dbl[])
                      n165 = Bundle(w356, w355) -> (w354:cluster{dbl[], dbl[]})  [unwired: 1 in]
                      n166 = Build Array(w354, w351) -> (w350:cluster{dbl[], dbl[]}[])
                      n167 = local write "I(B) 3"(w350) -> ()
                    }
                  }
                  n168 = local read "P(B)"() -> (w334:cluster{"yi":dbl[], dbl[]})
                  n169 = Unbundle(w334) -> ("yi"=w333:dbl[], w331:dbl[])
                  n170 = Build Array (concatenate)(w333, w332) -> (w329:dbl[])
                  n171 = Build Array (concatenate)(w331, w330) -> (w328:dbl[])
                  n172 = Bundle(w329, w328) -> (→"P(B)":cluster{dbl[], dbl[]})  [unwired: 1 in]
                }
                frame True {
                  # "Temperature plotting"
                  n173 = Quotient & Remainder(x=w383, y="Save Period") -> (x-y*floor(x/y)=w380:dbl)  [unwired: 1 out]
                  n174 = Greater?(x=w380, y=w381) -> (0:w379:bool)
                  n175 = case shown="True" w379 {
                    frame False {
                    }
                    frame True {
                      n176 = local write "Reset"(TRUE) -> ()
                    }
                  }
                  n177 = local read "Actual Temperature (K)"() -> (w366:dbl)
                  n178 = local read "Actual Current (pA)"() -> (w372:dbl)
                  n179 = local read "P(T)"() -> (w368:cluster{"yi":dbl[], dbl[]})
                  n180 = local read "I(T)"() -> (w378:cluster{dbl[], dbl[]})
                  n181 = Unbundle(w368) -> ("yi"=w369:dbl[], w365:dbl[])
                  n182 = Unbundle(w378) -> (w376:dbl[], w375:dbl[])
                  n183 = Build Array (concatenate)(w369, w366) -> (w370:dbl[])
                  n184 = Build Array (concatenate)(w365, w364) -> (w371:dbl[])
                  n185 = Build Array (concatenate)(w376, w366) -> (w374:dbl[])
                  n186 = Build Array (concatenate)(w375, w372) -> (w373:dbl[])
                  n187 = Bundle(w374, w373) -> (→"I(T)":cluster{dbl[], dbl[]})  [unwired: 1 in]
                  n188 = Bundle(w370, w371) -> (→"P(T)":cluster{dbl[], dbl[]})  [unwired: 1 in]
                }
              }
            }
            frame "Save" {
              n189 = local read "Temp/Magnetic Field"() -> (w387:bool)
              n190 = local read "Reset"() -> (w386:bool)
              n191 = Or(x=w386, y=w387) -> (x .or. y?=w385:bool)
              n192 = case shown="True" w385 {
                tunnel: w390 -> [w404 w406]
                tunnel: [w404 w409] -> w395
                tunnel: w389 -> [w403 w407]
                tunnel: [w403 w409] -> w394
                tunnel: w391 -> [w402 w408]
                tunnel: [w402 w409] -> w393
                tunnel: [w401 w409] -> w392
                tunnel: w388 -> [w401 w405]
                frame False {
                }
                frame True {
                  n193 = stacked-sequence {
                    tunnel: [_ _ w446] -> w409
                    tunnel: w408 -> [_ w435 _]
                    tunnel: w407 -> [w420 w433 _]
                    tunnel: w406 -> [w421 w434 _]
                    tunnel: w405 -> [_ w431 _]
                    frame #0 {
                      n194 = local read "B array"() -> (w411:dbl[])
                      n195 = local read "Counter"() -> (w419:i8)
                      n196 = local read "Averaged I(B)"() -> (w423:dbl[][])
                      n197 = local read "Up/Down"() -> (w422:bool)
                      n198 = call "Average_IB_curves.vi"("B array"=w411, "Up/Down"=w422, "Counter"=w419, "B in"=w421, "Averaged I(B) In"=w423, "I in"=w420) -> ("Averaged I(B) out"=w414:dbl[][])  [unwired: 5 in]
                      "Averaged I(B)" <- w414
                      n199 = Index Array(array=w414, index (row)=0 ("disabled index (col)")) -> (element=w412:dbl[])  [unwired: 1 in]
                      n200 = Index Array(array=w414, index (row)=1 ("disabled index (col)")) -> (element=w410:dbl[])  [unwired: 1 in]
                      n201 = Bundle("B array"=w411, "Averaged I(B) out"=w412) -> (w418:T6)  [unwired: 1 in]
                      n202 = Bundle("B array"=w411, "Averaged I(B) out"=w410) -> (w417:T6)  [unwired: 1 in]
                      n203 = Build Array(w418, w417) -> (→"I(B) /Averaged/ 2":T7)
                    }
                    frame #1 {
                      # "Save and Reset"
                      n204 = local read "Temp/Magnetic Field"() -> (w424:bool)
                      n205 = local read "Measurement File"() -> (w426:path)
                      n206 = local read "P(uC/mm^2)"() -> (w432:dbl[])
                      n207 = Build Array(w435, w434, w433, w431, w432) -> (w425:dbl[][])
                      n208 = case shown="False" w424 {
                        tunnel: w426 -> [_ _]
                        tunnel: w425 -> [w440 _]
                        frame False {
                          n209 = local read "Up/Down"() -> (w438:bool)
                          n210 = case shown="False" w438 {
                            tunnel: [w443 w444] -> w437
                            frame False {
                              n211 = local read "Measurement File_dn"() -> (w443:path)
                            }
                            frame True {
                              n212 = local read "Measurement File_up"() -> (w444:path)
                            }
                          }
                          n213 = call-poly <vilib>:"Write Delimited Spreadsheet.vi"("file path (dialog if empty)"=w437, "format (%.3f)"="%.5g", "2D data"=w440, "append to file? (F)"=TRUE ("transpose? (F)"), "transpose? (F)"=FALSE ("append to file? (F)")) -> ()  [unwired: 9 in, 2 out]
                        }
                        frame True {
                        }
                      }
                      n214 = case shown="True" "Reset IB?" {
                        frame False {
                        }
                        frame True {
                          n215 = local read "Up/Down"() -> (w445:bool)
                          n216 = case shown="False" w445 {
                            frame False {
                              n217 = invoke on="I(B) 3" class="XYGraph (strict)" method="Reinit To Default"() -> ()  [unwired: 3 in, 3 out]
                            }
                            frame True {
                            }
                          }
                        }
                      }
                      n218 = call-poly <vilib>:"Write Delimited Spreadsheet.vi"("file path (dialog if empty)"=w426, "format (%.3f)"="%.5g", "2D data"=w425, "append to file? (F)"=TRUE, "transpose? (F)"=TRUE) -> ()  [unwired: 9 in, 2 out]
                      n219 = local write "Reset"(FALSE ("Save")) -> ()
                    }
                    frame #2 {
                      w446 = dbl[] []
                      n220 = local write "P(uC/mm^2)"(w446) -> ()
                    }
                  }
                }
              }
            }
            frame "New" {
            }
          }
        }
      }
      frame Error {
        # "Return true for any case which should stop the loop."
      }
    }
  }
  n221 = while {
    shift-right: [w475] -> w44
    shift-left: w21 -> [w476]
    shift-right: [w477] -> w51
    shift-left: w52 -> [w478]
    tunnel: w47 -> [w474]
    tunnel: w46 -> [w473]
    tunnel: w24 -> [w472]
    tunnel: [w466] -> _
    tunnel: w31 -> [w465]
    tunnel: w19 -> [w464]
    stop <- "stop" stop-if-true
    n222 = event shown="[7] \"Sweep Field\": Value Change" {
      selector: _ -> [_ _ _ _ _ _ _ _ _ _ _ _ _ _ _]
      dyn-events: _ -> [_ _ _ _ _ _ _ _ _ _ _ _ _ _ _]
      timeout: 10 -> [_ _ _ _ _ _ _ _ _ _ _ _ _ _ _]
      tunnel: w478 -> [w488 w520 w529 w537 w548 w553 w557 w583 w599 _ w656 w673 w689 w699 w710]
      tunnel: [w487 w520 w529 w537 w548 w553 w557 w583 w599 _ w656 w673 w689 w699 w710] -> w477
      tunnel: w476 -> [w486 w519 w528 w538 w547 w555 w559 w584 w598 _ w657 w675 w693 w703 w712]
      tunnel: [w485 w519 w528 w538 w549 w555 w558 _ w598 _ w657 w674 w692 w702 w711] -> w475
      tunnel: w474 -> [w484 _ _ _ _ _ _ _ _ _ _ _ _ _ _]
      tunnel: w473 -> [w483 _ _ _ _ _ _ _ _ _ _ _ _ _ _]
      tunnel: w472 -> [w482 _ _ _ _ _ _ _ _ _ _ _ _ _ _]
      tunnel: [w480 w518 w527 w536 w550 w554 w556 w582 w597 _ w655 w672 w690 w700 _] -> w466
      tunnel: w465 -> [w480 w518 w530 w536 w550 w554 w556 w582 w597 _ w655 w672 w690 w700 _]
      tunnel: w464 -> [_ _ _ _ _ _ _ _ _ _ _ w676 w691 w704 w709]
      tunnel: [_ _ _ _ _ _ _ w584 _ _ _ _ _ _ _] -> _
      event Timeout {
        n223 = event-data() -> ()  [unwired: 1 in, 3 out]
        n224 = case shown="True" "Measuring" {
          tunnel: w488 -> [w490 w509]
          tunnel: [w490 w508] -> w487
          tunnel: w486 -> [w489 _]
          tunnel: [w489 w507] -> w485
          tunnel: w484 -> [_ w500]
          tunnel: w483 -> [_ w499]
          tunnel: w482 -> [_ w494]
          frame False {
          }
          frame True {
            w497 = ":FETCh? " ("data")
            w501 = u32 1000 ("byte count")
            # "Generate the data here."
            n225 = case shown="No Error" w494 {
              selector: w494 -> [w511 w512]
              tunnel: [w511 w512] -> w493
              tunnel: [w510 _] -> w492
              frame No Error {
                n226 = Get Date/Time In Seconds() -> (seconds since 1Jan1904=w510:timestamp)
              }
              frame Error {
              }
            }
            n227 = VISA Write(VISA resource name=w500, write buffer=w497, error in (no error)=w493) -> (VISA resource name out=w506:refnum<visa-resource-name>, error out=w504:errorcluster)  [unwired: 1 out]
            n228 = VISA Write(VISA resource name=w499, write buffer=w497, error in (no error)=w504) -> (VISA resource name out=w505:refnum<visa-resource-name>, error out=w503:errorcluster)  [unwired: 1 out]
            n229 = VISA Read(VISA resource name=w506, byte count=w501, error in (no error)=w503) -> (read buffer=w495:string, error out=w502:errorcluster)  [unwired: 2 out]
            n230 = VISA Read(VISA resource name=w505, byte count=w501, error in (no error)=w502) -> (read buffer=w496:string, error out=w498:errorcluster)  [unwired: 2 out]
            n231 = Bundle("seconds since 1Jan1904"=w492, "read buffer"=w495, "read buffer"=w496) -> (w491:T5)  [unwired: 1 in]
            n232 = Enqueue Element(queue=w509, element=w491, error in (no error)=w498) -> (queue out=w508:refnum<queue>, error out=w507:errorcluster)  [unwired: 1 in, 1 out]
          }
        }
      }
      event "Max Field (T)": Value Change {
        n233 = event-data() -> ()  [unwired: 1 in, 6 out]
        n234 = Divide(x="Max Field (T)", y="dB (T)") -> (x/y=w515:dbl)
        n235 = for {
          N: w515 -> [_]
          tunnel: "dB (T)" -> [w525]
          tunnel: [w522] -> w514 mode=indexing
          tunnel: "Min Field (T)" -> [w523]
          tunnel: [0.0] -> _ mode=indexing
          i -> [w526]
          n236 = Multiply(x=w526, y=w525) -> (x*y=w524:dbl)
          n237 = Add(x=w524, y=w523) -> (x+y=w522:dbl)
        }
        "B array" <- w514
      }
      event "Sweep Rate (T/min)": Value Change {
        n238 = event-data() -> ("NewVal"=w534:dbl)  [unwired: 1 in, 5 out]
        n239 = Number To Fractional String(number=w534, precision (6)=i16 3) -> (F-format string=w532:string)  [unwired: 2 in]
        n240 = Concatenate Strings("T" ("format string"), w532) -> (w531:string)
        n241 = call "GPIB - BusCommand.vi"("Command"=w531, "Address"=w530) -> ("Address(thru)"=w527:T4)  [unwired: 1 out]
      }
      event "Field To Zero": Value Change {
        n242 = event-data() -> ()  [unwired: 1 in, 6 out]
        n243 = Two Button Dialog(message="Do you want to switch off the field?", 1:"No" ("F button name (\"Cancel\")"), 2:"Yes" ("T button name (\"OK\")")) -> (T button?=w542:bool)
        n244 = case shown="True" w542 {
          tunnel: w536 -> [_ w545]
          frame False {
          }
          frame True {
            n245 = local read "Sweep Rate (T/min)"() -> (w544:dbl)
            n246 = call "ips_switchHeaterOff.vi"("Instrument address"=w545, "Rate"=w544) -> ("B"=w543:dbl)
            n247 = local write "Actual Field (T)"(w543) -> ()
          }
        }
      }
      event "Go to Set": Value Change {
        n248 = event-data() -> ()  [unwired: 1 in, 6 out]
        n249 = call "Set_B.vi"("error in (no error)"=w547, "address string"="25", "Set Field (T)"="Set Field (T)") -> ("error out"=w549:errorcluster)  [unwired: 8 in]
      }
      event "Measure /Pause": Value Change {
        n250 = event-data() -> ("NewVal"=w552:bool)  [unwired: 1 in, 5 out]
        n251 = local write "Measuring"(w552) -> ()
      }
      event "Stop": Value Change {
        n252 = event-data() -> ()  [unwired: 1 in, 6 out]
        n253 = local read "Measuring"() -> (w560:bool)
        n254 = case shown="True" w560 {
          tunnel: w559 -> [w561 w564]
          tunnel: [w561 w563] -> w558
          frame False {
          }
          frame True {
            w562 = FALSE ("Measuring")
            n255 = local read "SaveSweep"() -> (w567:bool)
            n256 = local write "Measuring"(w562) -> ()
            n257 = local read "Set Field (T)"() -> (w565:dbl)
            n258 = local write "Measure /Pause"(w562) -> ()
            n259 = case shown="True" w567 {
              frame False {
              }
              frame True {
                n260 = local read "Measurement File_average"() -> (w578:path)
                n261 = local read "I(B) /Averaged/ 2"() -> (w577:cluster{"B array":dbl[], dbl[]}[])
                n262 = Index Array(array=w577, index=0) -> (element=w574:cluster{"B array":dbl[], dbl[]})
                n263 = Index Array(array=w577, index=1) -> (element=w573:cluster{"B array":dbl[], dbl[]})
                n264 = Unbundle(w574) -> ("B array"=w572:dbl[], w571:dbl[])
                n265 = Unbundle(w573) -> ("B array"=w570:dbl[], w569:dbl[])
                n266 = Build Array(w572, w571, w570, w569) -> (w568:dbl[][])
                n267 = call-poly <vilib>:"Write Delimited Spreadsheet.vi"("file path (dialog if empty)"=w578, "format (%.3f)"="%.5g", "2D data"=w568, "append to file? (F)"=TRUE ("transpose? (F)"), "transpose? (F)"=TRUE ("append to file? (F)")) -> ()  [unwired: 9 in, 2 out]
              }
            }
            n268 = call "Set_B.vi"("error in (no error)"=w564, "address string"="25", "Set Field (T)"=w565) -> ("error out"=w563:errorcluster)  [unwired: 8 in]
          }
        }
      }
      event "Sweep Field": Value Change {
        n269 = event-data() -> ("NewVal"=w585:bool)  [unwired: 1 in, 5 out]
        n270 = case shown="True" w585 {
          frame False {
          }
          frame True {
            n271 = local read "Measurement File"() -> (w586:path)
            n272 = Two Button Dialog(message="Do you want to create additional files for the sweeping measurements?" ("string"), 1:"No" ("F button name (\"Cancel\")"), 2:"Yes" ("T button name (\"OK\")")) -> (T button?=w588:bool)
            n273 = case shown="True" w588 {
              tunnel: w586 -> [_ w593]
              frame False {
                n274 = local write "SaveSweep"(FALSE ("SaveSweep")) -> ()
              }
              frame True {
                n275 = call "Create_sweep_files.vi"("Measurement File"=w593) -> ("Path 3"=→"Measurement File_dn":path, "Path 2"=→"Measurement File_up":path, "Path"=→"Measurement File_average":path)  [unwired: 8 in]
                "SaveSweep" <- TRUE
              }
            }
          }
        }
      }
      event "Measure Noise": Value Change {
        n276 = event-data() -> ("NewVal"=w600:bool)  [unwired: 1 in, 5 out]
        n277 = case shown="True" w600 {
          frame False {
          }
          frame True {
            n278 = local read "Gain (V/A)"() -> (w605:dbl)
            n279 = call "Noise_measurement.vi"("Gain (V/A)"=w605, "Cycles"="Cycles", "Lower Cut-Off"="Cut-Off Frequency", "minimum value"="minimum value", "Filter On"="Filter On", "maximum value"="maximum value", "physical channels"="physical channels", "rate"="Rate", "samples per channel"="Samples per channel") -> ("Current (pA) Filtered"=→"Current (pA) Filtered":waveform(dbl), "PSD (pA/Hz^1/2) Peaks Removed"=→"PSD (pA/Hz^1/2) Peaks Removed":cluster{"f0":dbl, "df":dbl, "magnitude":dbl[]}, "Current (pA)"=→"Current (pA)":dbl[], "PSD (pA/Hz^1/2)"=→"PSD (pA/Hz^1/2)":cluster{"f0":dbl, "df":dbl, "magnitude":dbl[]})  [unwired: 3 in]
          }
        }
      }
      event "Calibrate": Value Change {
        n280 = event-data() -> ()  [unwired: 1 in, 6 out]
        n281 = case shown="True" "Calibrate" {
          frame False {
          }
          frame True {
            w617 = dbl[] []
            n282 = while {
              shift-right: [w650] -> w615
              shift-left: dbl[][] [] -> [w649]
              shift-right: [w633] -> _
              shift-left: w617 -> [w645]
              shift-right: [w642] -> _
              shift-left: w617 -> [w644]
              shift-right: [w632] -> _
              shift-left: w617 -> [w643]
              shift-right: [w624] -> _
              shift-left: 0.0 ("Set Field out") -> [w623]
              stop <- w646 stop-if-true
              n283 = call "Calibtarion.vi"("Dwell Time (ms)"="Dwell Time (ms)", "V array in (V)"=w645, "I array in (A)"=w643, "Collected array in"=w649, "B array in (T)"=w644, "Set Field (T)"=w623, "dB"="dB") -> ("Best Linear Fit"=w634:dbl[], "appended array"=→"appended array":dbl[][], "slope"=→"B/V (T/V)":dbl, "V array out (V)"=w633:dbl[], "Boolean"=w648:bool, "I array out (A)"=w632:dbl[], "intercept 2"=→"I0 (A)":dbl, "Collected array out"=w650:dbl[][], "intercept"=→"B0 (T)":dbl, "B array Out"=w642:dbl[], "slope 2"=→"V/I (Ohm)":dbl, "Best Linear Fit 2"=w639:dbl[], "Set Field out"=w624:dbl)
              n284 = Bundle("I array out (A)"=w632, "V array out (V)"=w633) -> (w641:T8)  [unwired: 1 in]
              n285 = Bundle("I array out (A)"=w632, "Best Linear Fit"=w634) -> (w635:T9)  [unwired: 1 in]
              n286 = Bundle("V array out (V)"=w633, "B array Out"=w642) -> (w637:T10)  [unwired: 1 in]
              n287 = Bundle("V array out (V)"=w633, "Best Linear Fit 2"=w639) -> (w638:T11)  [unwired: 1 in]
              n288 = Or(x=w648, y="stop 2") -> (x .or. y?=w646:bool)
              n289 = Build Array(w641, w635) -> (→"V_I":T12)
              n290 = Build Array(w637, w638) -> (→"B_V":T13)
            }
            n291 = flat-sequence {
              tunnel: w615 -> [w621]
              frame #0 {
                n292 = Two Button Dialog(message="Do you want to save calibration file?") -> (T button?=w620:bool)  [unwired: 2 in]
                n293 = case shown="True" w620 {
                  tunnel: w621 -> [_ w622]
                  frame False {
                  }
                  frame True {
                    n294 = call-poly <vilib>:"Write Delimited Spreadsheet.vi"("2D data"=w622) -> ()  [unwired: 13 in, 2 out]
                  }
                }
              }
            }
          }
        }
      }
      event "New Measurement File": Value Change {
        n295 = event-data() -> ()  [unwired: 1 in, 6 out]
        n296 = local read "Sweep Field"() -> (w652:bool)
        n297 = Open/Create/Replace File(prompt="Please select measurement file\n", operation (0:open)=T3."replace or create with confirmation") -> (refnum out=w658:refnum<file>)  [unwired: 4 in, 2 out]
        n298 = local write "refnum out"(w658) -> ()
        n299 = Refnum to Path(1:w658) -> (0:w653:path)
        n300 = case shown="True" w652 {
          tunnel: w653 -> [_ w661]
          frame False {
          }
          frame True {
            n301 = Two Button Dialog(message="Do you want to create additional files for the sweeping measurements?" ("string"), 1:"No" ("F button name (\"Cancel\")"), 2:"Yes" ("T button name (\"OK\")")) -> (T button?=w663:bool)
            n302 = case shown="False" w663 {
              tunnel: w661 -> [_ w671]
              frame False {
                n303 = local write "SaveSweep"(FALSE ("SaveSweep")) -> ()
              }
              frame True {
                n304 = call "Create_sweep_files.vi"("Measurement File"=w671) -> ("Path 3"=w668:path, "Path 2"=w669:path, "Path"=w670:path)  [unwired: 8 in]
                n305 = local write "Measurement File_dn"(w668) -> ()
                n306 = local write "Measurement File_average"(w670) -> ()
                n307 = local write "Measurement File_up"(w669) -> ()
                n308 = local write "SaveSweep"(TRUE) -> ()
              }
            }
          }
        }
        n309 = local write "Measurement File"(w653) -> ()
        n310 = local write "Offset?"(FALSE ("Offset?")) -> ()
        n311 = local write "First?"(TRUE ("First?")) -> ()
      }
      event "Heater On/Off": Value Change {
        n312 = event-data() -> ()  [unwired: 1 in, 6 out]
        n313 = case shown="True" "Heater On/Off" {
          tunnel: w676 -> [w681 w687]
          tunnel: w675 -> [w679 w688]
          tunnel: [w678 w686] -> w674
          frame False {
            n314 = VISA Write(VISA resource name=w681, write buffer="RANGE,1,0", error in (no error)=w679) -> (error out=w678:errorcluster)  [unwired: 2 out]
          }
          frame True {
            n315 = Number To Decimal String(number="Heater Range") -> (decimal integer string=w684:string)  [unwired: 1 in]
            n316 = Concatenate Strings("RANGE,1," ("write buffer"), w684) -> (w682:string)
            n317 = VISA Write(VISA resource name=w687, write buffer=w682, error in (no error)=w688) -> (error out=w686:errorcluster)  [unwired: 2 out]
          }
        }
      }
      event "Set temperature (K)": Value Change {
        n318 = event-data() -> ()  [unwired: 1 in, 6 out]
        n319 = local read "Set temperature (K)"() -> (w694:dbl)
        n320 = Number To Fractional String(number=w694, precision (6)=i16 3) -> (F-format string=w697:string)  [unwired: 2 in]
        n321 = Concatenate Strings("SETP 1," ("write buffer"), w697) -> (w695:string)
        n322 = VISA Write(VISA resource name=w691, write buffer=w695, error in (no error)=w693) -> (error out=w692:errorcluster)  [unwired: 2 out]
      }
      event "Temp Ramping Rate (K/min)": Value Change {
        n323 = event-data() -> ()  [unwired: 1 in, 6 out]
        n324 = local read "Temp Ramping Rate (K/min)"() -> (w701:dbl)
        n325 = Number To Fractional String(number=w701, precision (6)=i16 1) -> (F-format string=w707:string)  [unwired: 2 in]
        n326 = Concatenate Strings("RAMP 1,1," ("string"), w707) -> (w706:string)
        n327 = VISA Write(VISA resource name=w704, write buffer=w706, error in (no error)=w703) -> (error out=w702:errorcluster)  [unwired: 2 out]
      }
      event "Heater Range": Value Change {
        n328 = event-data() -> ()  [unwired: 1 in, 6 out]
        n329 = local read "Heater On/Off"() -> (w713:bool)
        n330 = case shown="False" w713 {
          tunnel: w712 -> [w714 w719]
          tunnel: [w714 w718] -> w711
          tunnel: w709 -> [_ w717]
          frame False {
          }
          frame True {
            n331 = local read "Heater Range"() -> (w715:enum16{"Off", "Low", "Medium", "High"})
            n332 = Number To Decimal String(number=w715) -> (decimal integer string=w721:string)  [unwired: 1 in]
            n333 = Concatenate Strings("RANGE,1," ("write buffer"), w721) -> (w720:string)
            n334 = VISA Write(VISA resource name=w717, write buffer=w720, error in (no error)=w719) -> (error out=w718:errorcluster)  [unwired: 2 out]
          }
        }
      }
    }
    n335 = Reciprocal(x="Sampling rate (Hz)") -> (1/x=w470:dbl)
    n336 = Multiply(x=w470, y=1000.0) -> (x*y=w468:dbl)
    n337 = Wait Until Next ms Multiple(millisecond multiple=w468) -> ()  [unwired: 1 out]
  }
  n338 = local read "Max Field (T)"() -> (w6:dbl)
  n339 = local read "Min Field (T)"() -> (w8:dbl)
  n340 = local read "dB (T)"() -> (w7:dbl)
  n341 = Divide(x=w6, y=w7) -> (x/y=w9:dbl)
  n342 = for {
    N: w9 -> [_]
    tunnel: w7 -> [w726]
    tunnel: [w723] -> w5 mode=indexing
    tunnel: w8 -> [w724]
    tunnel: [0.0] -> _ mode=indexing
    i -> [w727]
    n343 = Multiply(x=w727, y=w726) -> (x*y=w725:dbl)
    n344 = Add(x=w725, y=w724) -> (x+y=w723:dbl)
  }
  n345 = local write "B array"(w5) -> ()
  n346 = local read "Lake Shore"() -> (w22:refnum<visa-resource-name>)
  n347 = local read "IV converter"() -> (w42:refnum<visa-resource-name>)
  n348 = local read "Magnetic Field"() -> (w41:refnum<visa-resource-name>)
  n349 = VISA Close(VISA resource name=w42, error in (no error)=w44) -> (error out=w45:errorcluster)
  n350 = VISA Close(VISA resource name=w41, error in (no error)=w45) -> (error out=w43:errorcluster)
  n351 = Release Queue(queue=w51, error in (no error)=w43) -> (error out=w37:errorcluster)  [unwired: 1 in, 2 out]
  n352 = Merge Errors(w37, w36) -> (w38:errorcluster)
  n353 = VISA Close(VISA resource name=w22, error in (no error)=w38) -> (error out=w35:errorcluster)
  n354 = local read "refnum out"() -> (w33:refnum<file>)
  n355 = Close File(refnum=w33, error in=w35) -> (error out=w34:errorcluster)  [unwired: 1 out]
  n356 = call <vilib>:"Simple Error Handler.vi"("error in (no error)"=w34) -> ()  [unwired: 4 in, 5 out]
